vi "Find Time Zero.vi"() -> ()   [LabVIEW 2020]
uses:
  <vilib>/Analysis/1siggen.llb/Ramp Pattern by Samples.vi
  <vilib>/Analysis/NI_AALBase.lvlib
  SMC100-DQMH/Libraries/SMC100/SMC100.lvlib
  OphirPM-DQMH/Libraries/Ophir Power Meter/Ophir Power Meter.lvlib
panel:
  in  "Readout Rate (Hz)":i32=10
  in  "Ophir Port":i16=4
  in  "Power Range":u16(ring) items=["1.00mJ", "200uJ", "20.0uJ", "2.00uJ"]
  in  "SMC 100 Port":u8=3
  in  "Samples to Average":i32
  in  "Start Button":bool
  out "XY Graph":cluster{"Delay Positions":dbl[], "power":dbl[]}(graph)
  in  "Steps":i32
  in  "End Position":dbl
  in  "Start Posistion":dbl
  in  "OK":bool
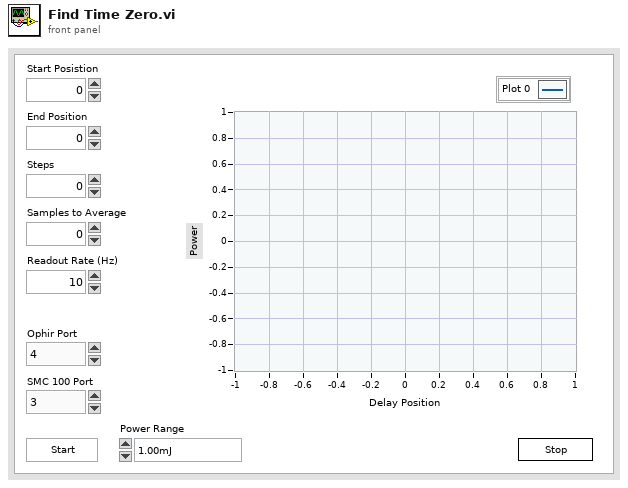
[diagram p1: front panel]
types:
  T1 = enum32{"Invalid", "Standard", "Closed", "Hidden", "Minimized", "Maximized"}
  T2 = enum32{"invalid app kind", "Development System", "Run Time System", "Student Edition", "Embedded LabVIEW", "Evaluation", "Custom"}
  T3 = cluster{"Core":cluster{"Current VI Reference":refnum<vi>, "Close Panel on Exit?":bool}, "Average":dbl[], "power":dbl[], "Delay Positions":dbl[], "Range Index":i32, "Step Index":i32}
  T4 = cluster{"Current VI Reference":refnum<vi>, "Close Panel on Exit?":bool}
  T5 = typedef "Ophir Power Meter.lvlib/Get Range Info (Reply Payload)--cluster.ctl" = cluster{"Range Info":cluster{"Strings Array":string[], "Symbols Array":i32[], "First Index":i32}, "Get Range Info_error":errorcluster}
  T6 = typedef "Ophir Power Meter.lvlib/Get Power Value (Reply Payload)--cluster.ctl" = cluster{"Power Value":dbl, "Get Power Value_error":errorcluster}
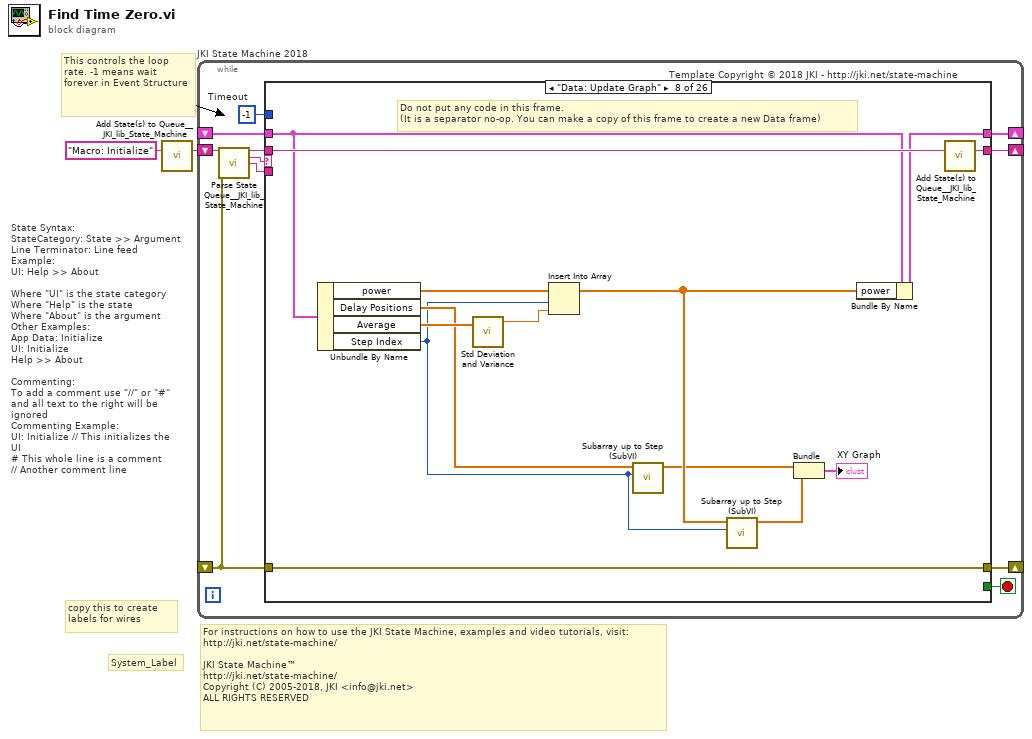
[diagram p0: block diagram]
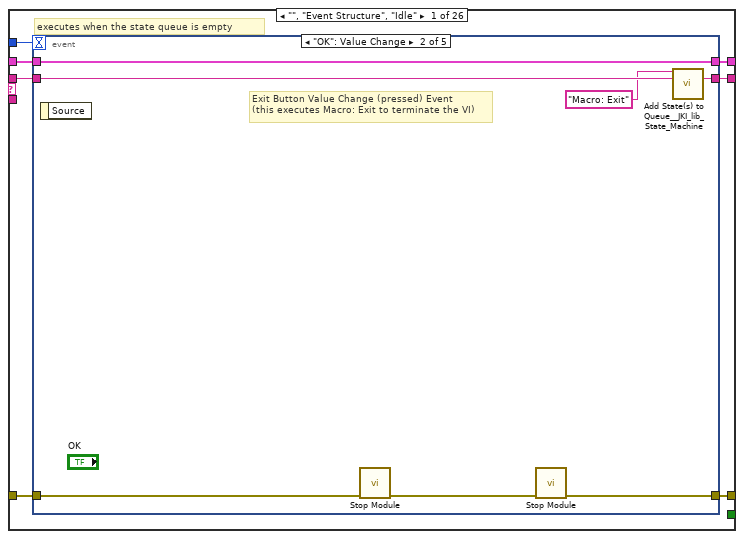
[diagram p2: hidden frame]
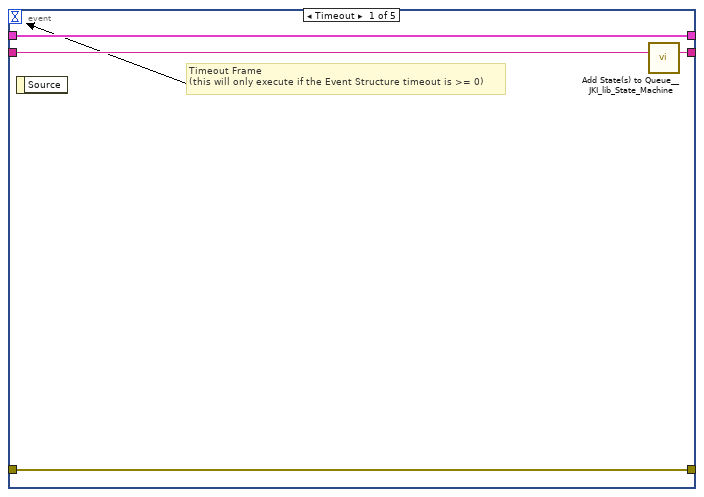
[diagram p3: hidden frame]
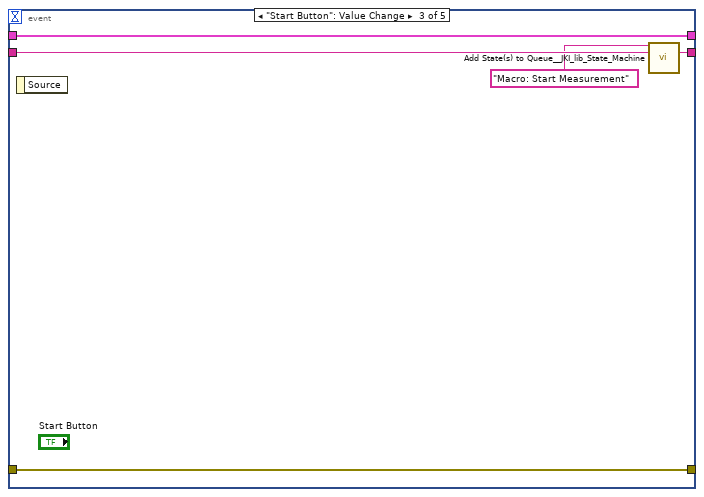
[diagram p4: hidden frame]
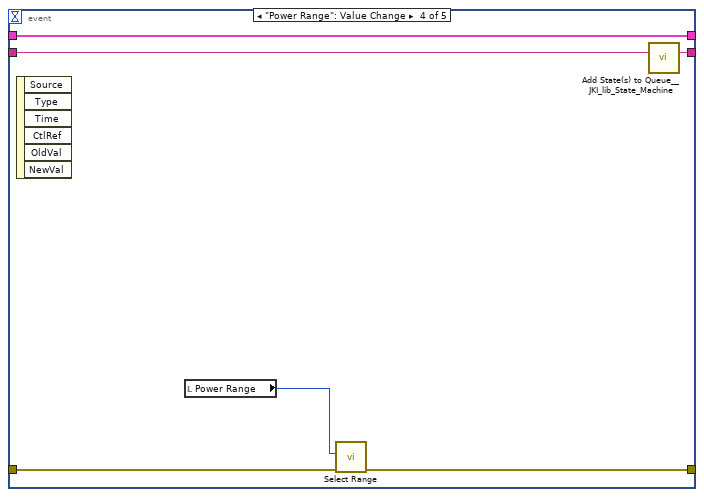
[diagram p5: hidden frame]
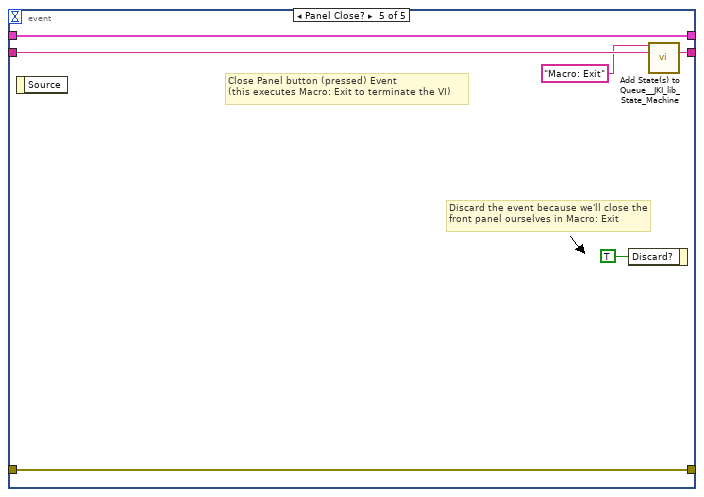
[diagram p6: hidden frame]
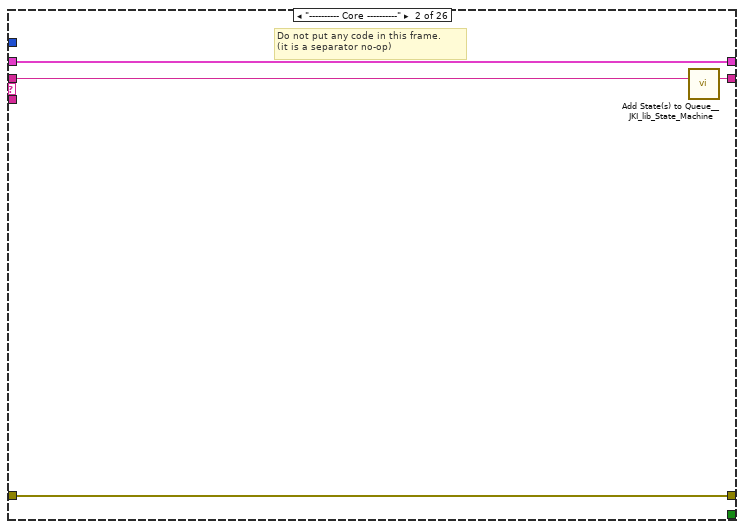
[diagram p7: hidden frame]
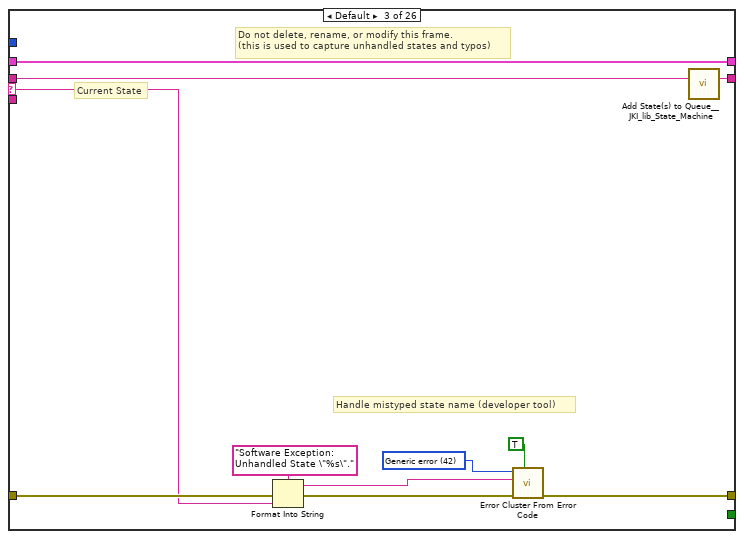
[diagram p8: hidden frame]
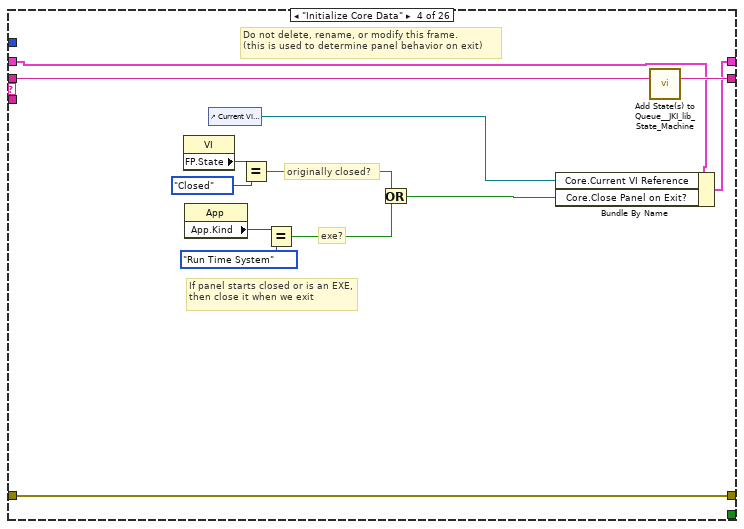
[diagram p9: hidden frame]
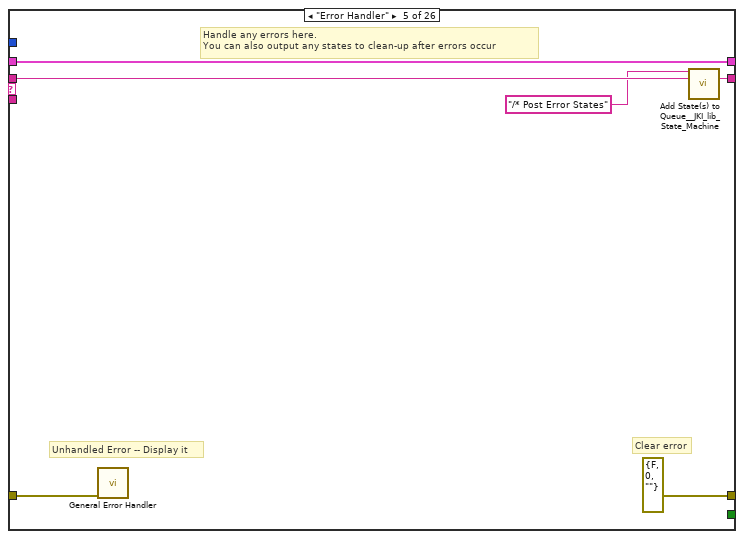
[diagram p10: hidden frame]
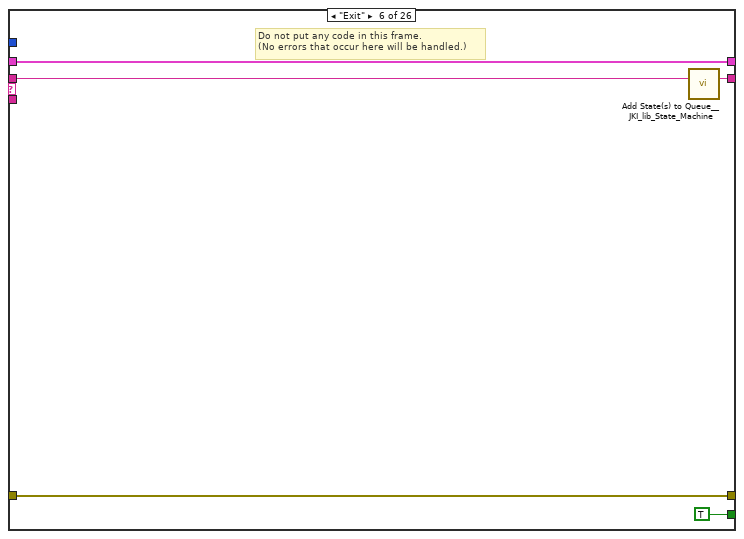
[diagram p11: hidden frame]
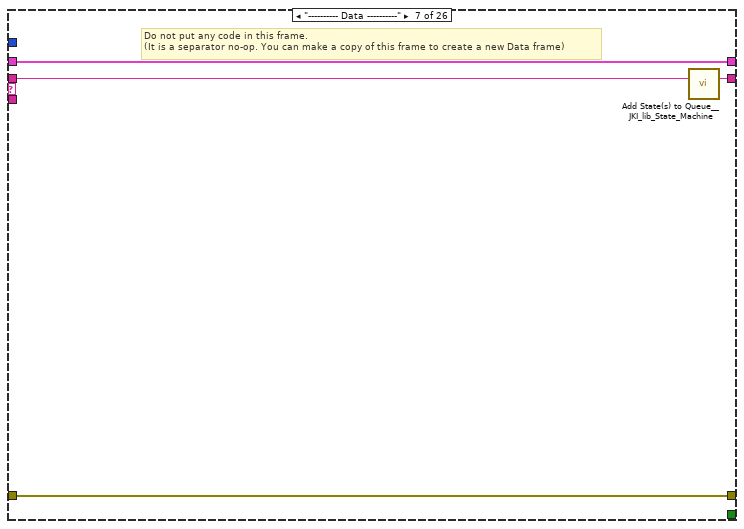
[diagram p12: hidden frame]
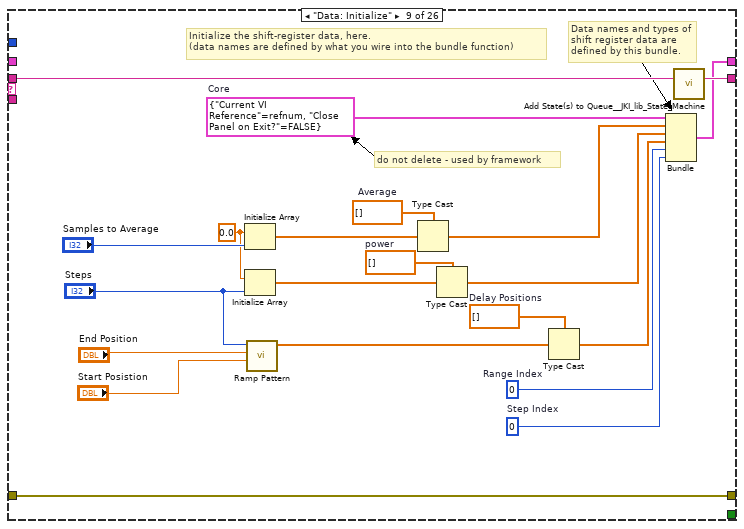
[diagram p13: hidden frame]
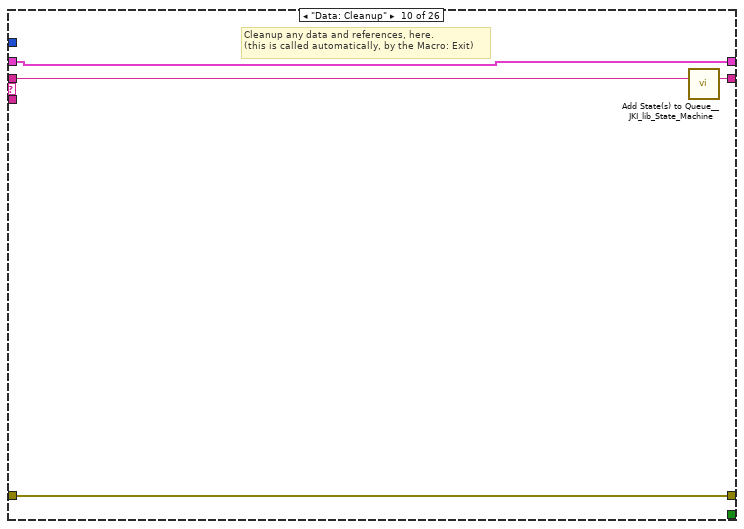
[diagram p14: hidden frame]
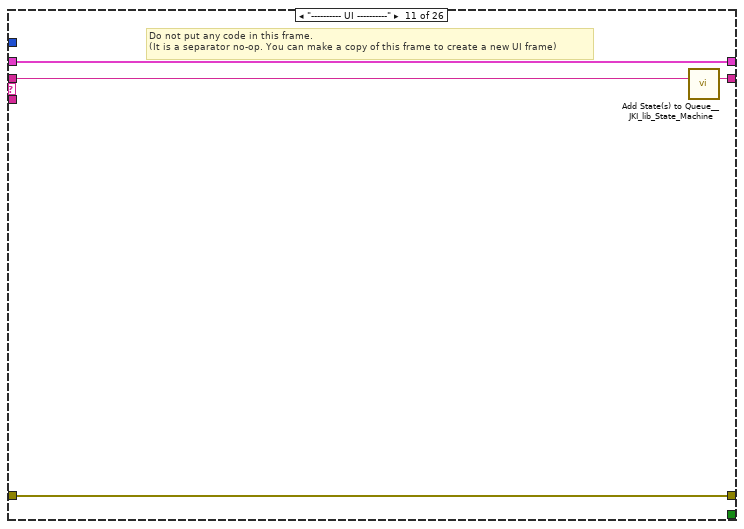
[diagram p15: hidden frame]
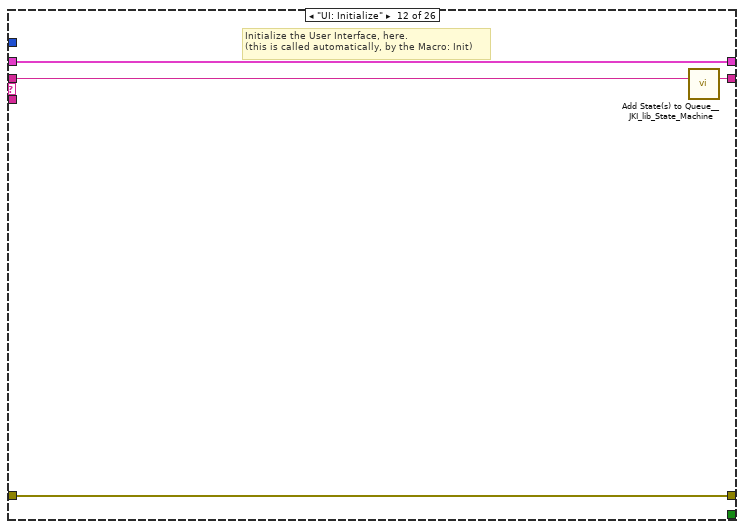
[diagram p16: hidden frame]
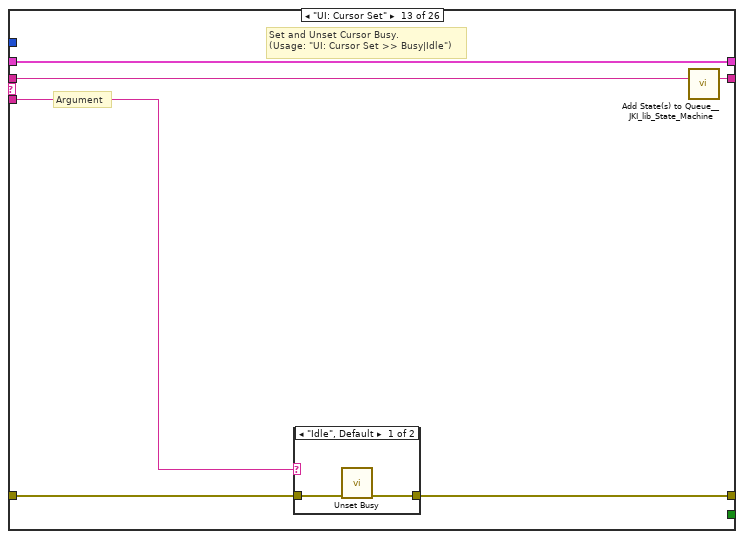
[diagram p17: hidden frame]
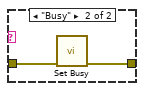
[diagram p18: hidden frame]
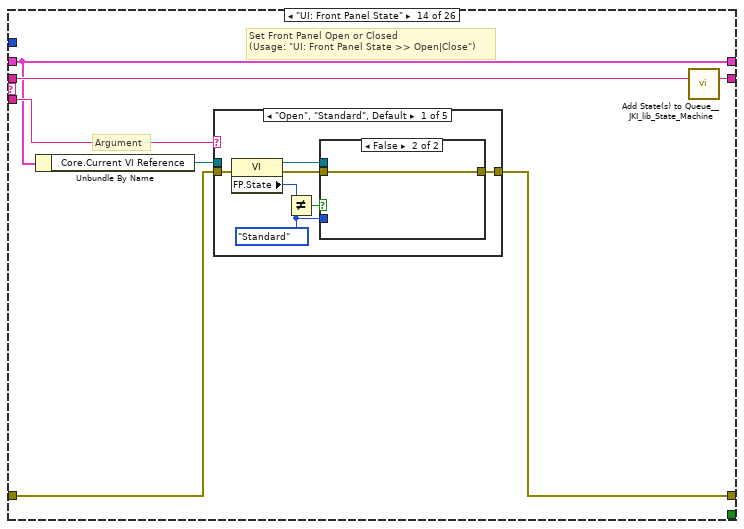
[diagram p19: hidden frame]
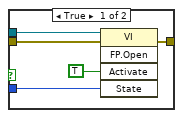
[diagram p20: hidden frame]
diagram:
  # "For instructions on how to use the JKI State Machine, examples and video tutorials, visit:\nhttp://jki.net/state-machine/\n\nJKI State Machine™\nhttp://jki.net/state-machine/\nCopyright (C) 2005-2018, JKI <info@jki.net>\nALL RIGHTS RESERVED"
  # "State Syntax:\nStateCategory: State >> Argument\nLine Terminator: Line feed\nExample:\nUI: Help >> About\n\nWhere \"UI\" is the state category\nWhere \"Help\" is the state\nWhere \"About\" is the argument\nOther Examples:\nApp Data: Initialize\nUI: Initialize\nHelp >> About\n\nCommenting:\nTo add a comment use \"//\" or \"#\" and all text to the right will be ignored\nCommenting Example:\nUI: Initialize // This initializes the UI\n# This whole line is a comment\n// Another comment line"
  # "copy this to create labels for wires"
  # "This controls the loop rate. -1 means wait forever in Event Structure"
  # "System_Label"
  n1 = call <vilib>:"Add State(s) to Queue__JKI_lib_State_Machine.vi"("State(s) in (\"\")"="Macro: Initialize") -> ("States Out"=w2:string)  [unwired: 14 in]
  n2 = while "JKI State Machine 2018" {
    shift-right: [w6] -> _
    shift-left: _ -> [w5]
    shift-right: [w9] -> _
    shift-left: _ -> [w3]
    shift-right: [w8] -> _
    shift-left: w2 -> [w10]
    stop <- w7 stop-if-true
    w4 = -1  # Timeout
    # "Template Copyright © 2018 JKI - http://jki.net/state-machine"
    n3 = call <vilib>:"Parse State Queue__JKI_lib_State_Machine.vi"("State Queue"=w10, "Error In (no error)"=w3) -> ("Remaining States"=w12:string, "Current State"=w13:string, "Arguments"=w11:string)  [unwired: 11 in]
    n4 = case shown="\"Data: Update Graph\"" w13 {
      selector: w13 -> [_ _ w53 _ _ _ _ _ _ _ _ _ _ _ _ _ _ _ _ _ _ _ _ _ _ _]
      tunnel: w12 -> [w20 w52 w57 w76 w82 w87 w91 w105 w126 w130 w134 w138 w144 w155 w219 w224 w229 w234 w244 w248 w255 w264 w274 w290 w308 w316]
      tunnel: w11 -> [_ _ _ _ _ _ _ _ _ _ _ _ w139 w150 _ _ _ _ _ _ _ _ _ _ _ _]
      tunnel: w5 -> [w18 w49 w55 w65 w79 w85 w88 w102 _ w127 w131 w136 w142 w149 w216 w221 w226 w231 w235 w245 w252 w261 w267 w288 w305 w312]
      tunnel: [w17 w50 w59 w74 errorcluster {"status"=FALSE, "code"=0, "source"=""} ("error out") w84 w89 w103 w124 w128 w132 w135 w140 w152 w217 w222 w227 w232 w242 w246 w251 w259 w272 w286 w304 w313] -> w9
      tunnel: w3 -> [w16 w50 w58 w74 w78 w84 w89 w103 w124 w128 w132 w135 w141 w153 w217 w222 w227 w232 w242 w246 w253 w262 w272 w287 w306 w314]
      tunnel: [w19 w51 w56 w75 w81 w86 w90 w104 w125 w129 w133 w137 w143 w154 w218 w223 w228 w233 w243 w247 w254 w263 w273 w289 w307 w315] -> w8
      tunnel: [_ _ _ _ _ TRUE _ _ _ _ _ _ _ _ _ _ _ _ _ _ _ _ _ _ _ _] -> w7
      tunnel: [w15 w49 w55 w64 w79 w85 w88 w101 w115 w127 w131 w136 w142 w149 w216 w221 w226 w231 w235 w245 w252 w261 w266 w288 w305 w312] -> w6
      tunnel: w4 -> [w14 _ _ _ _ _ _ _ _ _ _ _ _ _ _ _ _ _ _ _ _ _ _ _ _ _]
      frame "", "Event Structure", "Idle" {
        # "executes when the state queue is empty"
        n5 = event shown="[1] \"OK\": Value Change" {
          selector: _ -> [_ _ _ _ _]
          dyn-events: _ -> [_ _ _ _ _]
          timeout: w14 -> [_ _ _ _ _]
          tunnel: w20 -> [w24 w31 w36 w42 w48]
          tunnel: [w23 w30 w35 w41 w47] -> w19
          tunnel: w18 -> [w21 w28 w33 w39 w45]
          tunnel: [w22 w25 w34 w38 w46] -> w17
          tunnel: w16 -> [w22 w29 w34 w40 w46]
          tunnel: [w21 w28 w33 w39 w45] -> w15
          event Timeout {
            # "Timeout Frame\n(this will only execute if the Event Structure timeout is >= 0)"
            n6 = event-data() -> ()  [unwired: 1 in, 1 out]
            n7 = call <vilib>:"Add State(s) to Queue__JKI_lib_State_Machine.vi"("State(s) in (\"\")"=w24) -> ("States Out"=w23:string)  [unwired: 14 in]
          }
          event "OK": Value Change {
            # "Exit Button Value Change (pressed) Event\n(this executes Macro: Exit to terminate the VI)"
            n8 = event-data() -> ()  [unwired: 1 in, 1 out]
            n9 = call "Stop Module.vi"("error in (no error)"=w29) -> ("error out"=w26:errorcluster)  [unwired: 10 in]
            n10 = call "Stop Module.vi"("error in (no error)"=w26) -> ("error out"=w25:errorcluster)  [unwired: 10 in]
            n11 = call <vilib>:"Add State(s) to Queue__JKI_lib_State_Machine.vi"("State(s) in Front (\"\")"="Macro: Exit", "State(s) in (\"\")"=w31) -> ("States Out"=w30:string)  [unwired: 13 in]
          }
          event "Start Button": Value Change {
            n12 = event-data() -> ()  [unwired: 1 in, 1 out]
            n13 = call <vilib>:"Add State(s) to Queue__JKI_lib_State_Machine.vi"("State(s) in Front (\"\")"="Macro: Start Measurement", "State(s) in (\"\")"=w36) -> ("States Out"=w35:string)  [unwired: 13 in]
          }
          event "Power Range": Value Change {
            n14 = event-data() -> ()  [unwired: 1 in, 6 out]
            n15 = local read "Power Range"() -> (w37:u16)
            n16 = call "Select Range.vi"("error in (no error)"=w40, "Range Number"=w37) -> ("error out"=w38:errorcluster)  [unwired: 9 in]
            n17 = call <vilib>:"Add State(s) to Queue__JKI_lib_State_Machine.vi"("State(s) in (\"\")"=w42) -> ("States Out"=w41:string)  [unwired: 14 in]
          }
          event Panel Close? {
            # "Discard the event because we'll close the front panel ourselves in Macro: Exit"
            # "Close Panel button (pressed) Event\n(this executes Macro: Exit to terminate the VI)"
            n18 = event-data() -> ()  [unwired: 1 in, 1 out]
            n19 = event-data("Discard?"=TRUE) -> ()  [unwired: 1 in, 1 out]
            n20 = call <vilib>:"Add State(s) to Queue__JKI_lib_State_Machine.vi"("State(s) in Front (\"\")"="Macro: Exit", "State(s) in (\"\")"=w48) -> ("States Out"=w47:string)  [unwired: 13 in]
          }
        }
      }
      frame "---------- Core ----------" {
        # "Do not put any code in this frame.\n(it is a separator no-op)"
        n21 = call <vilib>:"Add State(s) to Queue__JKI_lib_State_Machine.vi"("State(s) in (\"\")"=w52) -> ("States Out"=w51:string)  [unwired: 14 in]
      }
      frame Default {
        w62 = 42 items=["No error", "Argument error", "Memory is full", "Out of zone", "End of file", "File already open", "Generic file I/O error", "File not found", "File permission error", "Disk is full", "Duplicate path", "Too many files open", "System feature not enabled", "Resource file not found", "Cannot add resource", "Resource not found", "Image not found", "Image memory error", "Pen does not exist", "Config type invalid", "Config token not found", "Config parse error", "Config memory error", "Bad external code format", "Bad external code offset", "External code not present", "Null window", "Destroy window error", "Null menu", "Print aborted", "Bad print record", "Print driver error", "Windows error during printing", "Memory error during printing", "Print dialog error", "Generic print error", "Invalid device refnum", "Device not found", "Device parameter error", "Device unit error", "Cannot open device", "Device call aborted", "Generic error", "Cancelled by user", "Object ID too low", "Object ID too high", "Object not in heap", "Unknown heap", "Unknown object (invalid DefProc)", "Unknown object (DefProc not in table)", "Message out of range", "Invalid (null) method", "Unknown message", "Manager call not supported", "Bad address", "Network operation in progress", "Network operation timed out", "Connection is busy", "Network attribute not supported", "Network error", "Address in use", "System out of memory", "Connection aborted", "Connection refused", "Not connected", "Already connected", "Connection closed", "Initialization error (interapplication manager)", "Bad occurrence", "Wait on unbound occurrence handler", "Occurrence queue overflow", "Datalog type conflict", "Unused", "Unrecognized type (interapplication manager)", "Memory corrupt", "Failed to make temporary DLL", "Old CIN version", "Drag socket not found", "Failed to load drop-object", "Failed to register OLE object", "Failed to release OLE object", "Format specifier type mismatch", "Unknown format specifier", "Too few format specifiers", "Too many format specifiers", "Scan failed", "Newer CIN version", "Error converting to variant", "Runtime menu error", "Password tampered", "Variant attribute not found", "Incompatible variant data type", "Event data is not available", "Event Store is not present", "Occurrence is not found", "Event Queue is not created", "Event info is not available", "Refnum passed is NULL", "Error retrieving Class GUID", "Error retrieving CoClass GUID", "Error retrieving TypeLib GUID.", "Bad built application magic bytes.", "Specific driver is different from the specific driver associated with the Logical Name.", "There is no session opened to the class driver.", "Max Error", "MAX - Error with config objects", "MAX - Error loading configuration", "MAX - Group not supported"]
        # "Current State"
        # "Do not delete, rename, or modify this frame.\n(this is used to capture unhandled states and typos)"
        # "Handle mistyped state name (developer tool)"
        n22 = Format Into String(format string="Software Exception: Unhandled State \"%s\"." ("message"), error in=w58, w53) -> (resulting string=w61:string, error out=w60:errorcluster)  [unwired: 1 in]
        n23 = call <vilib>:"Error Cluster From Error Code.vi"("show call chain? (False)"=TRUE, "error in (no error)"=w60, "error message (\"\")"=w61, "error code (0)"=w62) -> ("error out"=w59:errorcluster)  [unwired: 5 in]
        n24 = call <vilib>:"Add State(s) to Queue__JKI_lib_State_Machine.vi"("State(s) in (\"\")"=w57) -> ("States Out"=w56:string)  [unwired: 14 in]
      }
      frame "Initialize Core Data" {
        # "Do not delete, rename, or modify this frame.\n(this is used to determine panel behavior on exit)"
        # "originally closed?"
        # "exe?"
        # "If panel starts closed or is an EXE, then close it when we exit"
        n25 = property class="VI"() -> ("FP.State"=w68:T1)  [unwired: 2 in, 2 out]
        n26 = property class="App"() -> ("App.Kind"=w73:T2)  [unwired: 2 in, 2 out]
        n27 = control-ref of="Current VI Reference"() -> (w69:refnum<vi>)
        n28 = Equal?(x=w68, y=T1."Closed" ("Front Panel Window:State")) -> (x = y?=w66:bool)
        n29 = Equal?(x=w73, y=T2."Run Time System" ("Application:Kind")) -> (x = y?=w71:bool)
        n30 = Or(x=w66, y=w71) -> (x .or. y?=w70:bool)
        n31 = Bundle By Name(cluster=w65, "Core.Current VI Reference"=w69, "Core.Close Panel on Exit?"=w70) -> (w64:T3)
        n32 = call <vilib>:"Add State(s) to Queue__JKI_lib_State_Machine.vi"("State(s) in (\"\")"=w76) -> ("States Out"=w75:string)  [unwired: 14 in]
      }
      frame "Error Handler" {
        # "Unhandled Error -- Display it"
        # "Handle any errors here.\nYou can also output any states to clean-up after errors occur"
        # "Clear error"
        n33 = call <vilib>:"General Error Handler.vi"("error in (no error)"=w78) -> ()  [unwired: 10 in, 5 out]
        n34 = call <vilib>:"Add State(s) to Queue__JKI_lib_State_Machine.vi"("State(s) in Front (\"\")"="/* Post Error States", "State(s) in (\"\")"=w82) -> ("States Out"=w81:string)  [unwired: 13 in]
      }
      frame "Exit" {
        # "Do not put any code in this frame.\n(No errors that occur here will be handled.)"
        n35 = call <vilib>:"Add State(s) to Queue__JKI_lib_State_Machine.vi"("State(s) in (\"\")"=w87) -> ("States Out"=w86:string)  [unwired: 14 in]
      }
      frame "---------- Data ----------" {
        # "Do not put any code in this frame.\n(It is a separator no-op. You can make a copy of this frame to create a new Data frame)"
        n36 = call <vilib>:"Add State(s) to Queue__JKI_lib_State_Machine.vi"("State(s) in (\"\")"=w91) -> ("States Out"=w90:string)  [unwired: 14 in]
      }
      frame "Data: Update Graph" {
        # "Do not put any code in this frame.\n(It is a separator no-op. You can make a copy of this frame to create a new Data frame)"
        n37 = Unbundle By Name(w102) -> ("power"=w99:dbl[], "Delay Positions"=w96:dbl[], "Average"=w100:dbl[], "Step Index"=w92:i32)
        n38 = call <vilib>:"Std Deviation and Variance.vi"("X"=w100) -> ("mean"=w98:dbl)  [unwired: 1 in, 2 out]
        n39 = Insert Into Array(array=w99, index=w92, new element=w98) -> (w95:dbl[])
        n40 = call "Subarray up to Step (SubVI).vi"("Step Index"=w92, "Delay Positions"=w96) -> ("Array"=w94:dbl[])  [unwired: 9 in]
        n41 = call "Subarray up to Step (SubVI).vi"("Step Index"=w92, "Delay Positions"=w95) -> ("Array"=w93:dbl[])  [unwired: 9 in]
        n42 = Bundle("Array"=w94, "Array"=w93) -> (→"XY Graph":cluster{"Array":dbl[], "Array":dbl[]})  [unwired: 1 in]
        n43 = Bundle By Name(cluster=w102, "power"=w95) -> (w101:T3)
        n44 = call <vilib>:"Add State(s) to Queue__JKI_lib_State_Machine.vi"("State(s) in (\"\")"=w105) -> ("States Out"=w104:string)  [unwired: 14 in]
      }
      frame "Data: Initialize" {
        w106 = dbl[] []  # Delay Positions
        w108 = dbl[] []  # power
        w110 = dbl[] []  # Average
        w113 = 0  # Step Index
        w114 = 0  # Range Index
        w121 = 0.0 ("element")
        w123 = T4 {"Current VI Reference"=refnum, "Close Panel on Exit?"=FALSE}  # Core
        # "do not delete - used by framework"
        # "Data names and types of shift register data are defined by this bundle."
        # "Initialize the shift-register data, here.\n(data names are defined by what you wire into the bundle function)"
        n45 = Initialize Array(w121, "Samples to Average") -> (w112:dbl[])
        n46 = Initialize Array(w121, "Steps") -> (w120:dbl[])
        n47 = call-poly <vilib>:"Ramp Pattern.vi"("start"="Start Posistion", "end"="End Position", "samples"="Steps") -> ("Ramp Pattern"=w116:dbl[])  [unwired: 7 in, 1 out]
        n48 = Type Cast(type=w110, x=w112) -> (*(type *) &x=w111:dbl[])
        n49 = Type Cast(type=w108, x=w120) -> (*(type *) &x=w109:dbl[])
        n50 = Type Cast(type=w106, x=w116) -> (*(type *) &x=w107:dbl[])
        n51 = Bundle("Core"=w123, "Average"=w111, "power"=w109, "Delay Positions"=w107, "Range Index"=w114, "Step Index"=w113) -> (w115:T3)  [unwired: 1 in]
        n52 = call <vilib>:"Add State(s) to Queue__JKI_lib_State_Machine.vi"("State(s) in (\"\")"=w126) -> ("States Out"=w125:string)  [unwired: 14 in]
      }
      frame "Data: Cleanup" {
        # "Cleanup any data and references, here.\n(this is called automatically, by the Macro: Exit)"
        n53 = call <vilib>:"Add State(s) to Queue__JKI_lib_State_Machine.vi"("State(s) in (\"\")"=w130) -> ("States Out"=w129:string)  [unwired: 14 in]
      }
      frame "---------- UI ----------" {
        # "Do not put any code in this frame.\n(It is a separator no-op. You can make a copy of this frame to create a new UI frame)"
        n54 = call <vilib>:"Add State(s) to Queue__JKI_lib_State_Machine.vi"("State(s) in (\"\")"=w134) -> ("States Out"=w133:string)  [unwired: 14 in]
      }
      frame "UI: Initialize" {
        # "Initialize the User Interface, here.\n(this is called automatically, by the Macro: Init)"
        n55 = call <vilib>:"Add State(s) to Queue__JKI_lib_State_Machine.vi"("State(s) in (\"\")"=w138) -> ("States Out"=w137:string)  [unwired: 14 in]
      }
      frame "UI: Cursor Set" {
        # "Argument"
        # "Set and Unset Cursor Busy.\n(Usage: \"UI: Cursor Set >> Busy|Idle\")"
        n56 = case shown="\"Idle\", Default" w139 {
          tunnel: w141 -> [w146 w148]
          tunnel: [w145 w147] -> w140
          frame "Idle", Default {
            n57 = call <vilib>:"Unset Busy.vi"("error in (no error)"=w146) -> ("error out"=w145:errorcluster)  [unwired: 10 in]
          }
          frame "Busy" {
            n58 = call <vilib>:"Set Busy.vi"("error in (no error)"=w148) -> ("error out"=w147:errorcluster)  [unwired: 9 in, 1 out]
          }
        }
        n59 = call <vilib>:"Add State(s) to Queue__JKI_lib_State_Machine.vi"("State(s) in (\"\")"=w144) -> ("States Out"=w143:string)  [unwired: 14 in]
      }
      frame "UI: Front Panel State" {
        # "Argument"
        # "Set Front Panel Open or Closed\n(Usage: \"UI: Front Panel State >> Open|Close\")"
        n60 = Unbundle By Name(w149) -> ("Core.Current VI Reference"=w151:refnum<vi>)
        n61 = case shown="\"Open\", \"Standard\", Default" w150 {
          tunnel: w153 -> [w161 w174 w185 w197 w209]
          tunnel: [w162 w175 w186 w198 w210] -> w152
          tunnel: w151 -> [_ _ _ _ _]
          frame "Open", "Standard", Default {
            w156 = T1."Standard" ("State")
            n62 = property class="VI"(error in=w161) -> (reference out=w159:refnum<vi>, error out=w160:errorcluster, "FP.State"=w158:T1)  [unwired: 1 in]
            n63 = Not Equal?(x=w158, y=w156) -> (x != y?=w157:bool)
            n64 = case shown="False" w157 {
              tunnel: [w166 w168] -> w162
              tunnel: w160 -> [w165 w168]
              tunnel: w159 -> [w164 _]
              tunnel: w156 -> [w163 _]
              frame True {
                n65 = invoke class="VI" method="FP.Open"(reference=w164, error in=w165, "Activate"=TRUE, "State"=w163) -> (error out=w166:errorcluster)  [unwired: 1 in, 4 out]
              }
              frame False {
              }
            }
          }
          frame "Close", "Closed" {
            n66 = property class="VI"(error in=w174) -> (reference out=w172:refnum<vi>, error out=w173:errorcluster, "FP.State"=w170:T1)  [unwired: 1 in]
            n67 = Not Equal?(x=w170, y=T1."Closed" ("Front Panel Window:State")) -> (x != y?=w169:bool)
            n68 = case shown="True" w169 {
              tunnel: [w176 w179] -> w175
              tunnel: w173 -> [w176 w178]
              tunnel: w172 -> [_ w177]
              frame False {
              }
              frame True {
                n69 = invoke class="VI" method="FP.Close"(reference=w177, error in=w178) -> (error out=w179:errorcluster)  [unwired: 1 in, 2 out]
              }
            }
          }
          frame "Hidden", "Hide" {
            w180 = T1."Hidden" ("State")
            n70 = property class="VI"(error in=w185) -> (reference out=w183:refnum<vi>, error out=w184:errorcluster, "FP.State"=w182:T1)  [unwired: 1 in]
            n71 = Not Equal?(x=w182, y=w180) -> (x != y?=w181:bool)
            n72 = case shown="True" w181 {
              tunnel: [w190 w191] -> w186
              tunnel: w184 -> [w189 w191]
              tunnel: w183 -> [w188 _]
              tunnel: w180 -> [w187 _]
              frame True {
                n73 = invoke class="VI" method="FP.Open"(reference=w188, error in=w189, "State"=w187) -> (error out=w190:errorcluster)  [unwired: 2 in, 4 out]
              }
              frame False {
              }
            }
          }
          frame "Minimize", "Minimized" {
            w192 = T1."Minimized" ("State")
            n74 = property class="VI"(error in=w197) -> (reference out=w195:refnum<vi>, error out=w196:errorcluster, "FP.State"=w194:T1)  [unwired: 1 in]
            n75 = Not Equal?(x=w194, y=w192) -> (x != y?=w193:bool)
            n76 = case shown="True" w193 {
              tunnel: [w202 w203] -> w198
              tunnel: w196 -> [w201 w203]
              tunnel: w195 -> [w200 _]
              tunnel: w192 -> [w199 _]
              frame True {
                n77 = invoke class="VI" method="FP.Open"(reference=w200, error in=w201, "State"=w199) -> (error out=w202:errorcluster)  [unwired: 2 in, 4 out]
              }
              frame False {
              }
            }
          }
          frame "Maximize", "Maximized" {
            w204 = T1."Maximized" ("State")
            n78 = property class="VI"(error in=w209) -> (reference out=w207:refnum<vi>, error out=w208:errorcluster, "FP.State"=w206:T1)  [unwired: 1 in]
            n79 = Not Equal?(x=w206, y=w204) -> (x != y?=w205:bool)
            n80 = case shown="True" w205 {
              tunnel: [w214 w215] -> w210
              tunnel: w208 -> [w213 w215]
              tunnel: w207 -> [w212 _]
              tunnel: w204 -> [w211 _]
              frame True {
                n81 = invoke class="VI" method="FP.Open"(reference=w212, error in=w213, "State"=w211) -> (error out=w214:errorcluster)  [unwired: 2 in, 4 out]
              }
              frame False {
              }
            }
          }
        }
        n82 = call <vilib>:"Add State(s) to Queue__JKI_lib_State_Machine.vi"("State(s) in (\"\")"=w155) -> ("States Out"=w154:string)  [unwired: 14 in]
      }
      frame "---------- Macro ----------" {
        # "Do not put any code in this frame.\n(It is a separator no-op. You can make a copy of this frame to create a new Macro frame)"
        n83 = call <vilib>:"Add State(s) to Queue__JKI_lib_State_Machine.vi"("State(s) in (\"\")"=w219) -> ("States Out"=w218:string)  [unwired: 14 in]
      }
      frame "Macro: Measurement Cycle" {
        # "Do not put any code in this frame.\n(It is a separator no-op. You can make a copy of this frame to create a new Macro frame)"
        n84 = call <vilib>:"Add State(s) to Queue__JKI_lib_State_Machine.vi"("State(s) in (\"\")"=w224, "State(s) at Back (\"\")"="Devices: Move to Position\nDevices: Get Average Power\nData: Update Graph\nDevices: Finished?" ("State(s) at Back (\"\")")) -> ("States Out"=w223:string)  [unwired: 13 in]
      }
      frame "Macro: Start Measurement" {
        # "Do not put any code in this frame.\n(It is a separator no-op. You can make a copy of this frame to create a new Macro frame)"
        n85 = call <vilib>:"Add State(s) to Queue__JKI_lib_State_Machine.vi"("State(s) in (\"\")"=w229, "State(s) at Back (\"\")"="Data: Initialize\nDevices: Initialize\nMacro: Measurement Cycle" ("State(s) at Back (\"\")")) -> ("States Out"=w228:string)  [unwired: 13 in]
      }
      frame "Macro: Initialize" {
        # "Initialization Macro\n(This is called once, when the VI starts)"
        n86 = call <vilib>:"Add State(s) to Queue__JKI_lib_State_Machine.vi"("State(s) in Front (\"\")"="Devices: Start\nData: Initialize\nInitialize Core Data\nUI: Initialize\nUI: Front Panel State >> Open\nDevices: Get Ranges", "State(s) in (\"\")"=w234) -> ("States Out"=w233:string)  [unwired: 13 in]
      }
      frame "Macro: Exit" {
        # "Exit Macro\n(This is called once, when the VI exits)"
        n87 = Unbundle By Name(w235) -> ("Core.Close Panel on Exit?"=w236:bool)
        n88 = Select(t="UI: Front Panel State >> Close", s=w236, f="") -> (s? t:f=w239:string)
        n89 = call <vilib>:"Add State(s) to Queue__JKI_lib_State_Machine.vi"("State(s) in (\"\")"=w239, "State(s) at Back (\"\")"="Data: Cleanup\nExit") -> ("States Out"=w237:string)  [unwired: 13 in]
        n90 = call <vilib>:"Add State(s) to Queue__JKI_lib_State_Machine.vi"("State(s) in Front (\"\")"=w237, "State(s) in (\"\")"=w244) -> ("States Out"=w243:string)  [unwired: 13 in]
      }
      frame "---------- Devices ----------" {
        # "Template Separator\n(You can make a copy of, or modify, this frame)"
        n91 = call <vilib>:"Add State(s) to Queue__JKI_lib_State_Machine.vi"("State(s) in (\"\")"=w248) -> ("States Out"=w247:string)  [unwired: 14 in]
      }
      frame "Devices: Get Ranges" {
        # "Template Separator\n(You can make a copy of, or modify, this frame)"
        n92 = call "Get Range Info.vi"("error in (no error)"=w253) -> ("error out"=w251:errorcluster, "Reply Payload"=w250:T5)  [unwired: 8 in, 1 out]
        n93 = Unbundle By Name(w250) -> ("Range Info.Strings Array"=w249:string[])
        n94 = property on="Power Range" class="Ring (strict)"("Strings []"=w249) -> ()  [unwired: 2 in, 2 out]
        n95 = call <vilib>:"Add State(s) to Queue__JKI_lib_State_Machine.vi"("State(s) in (\"\")"=w255) -> ("States Out"=w254:string)  [unwired: 14 in]
      }
      frame "Devices: Start" {
        # "Give devices time to initialize"
        # "Template Separator\n(You can make a copy of, or modify, this frame)"
        n96 = call "Start Module.vi"("error in (no error)"=w262, "Port Number"="Ophir Port") -> ("error out"=w260:errorcluster)  [unwired: 6 in, 3 out]
        n97 = Wait (ms)(milliseconds to wait=u32 2000) -> ()  [unwired: 1 out]
        n98 = call "Start Module.vi"("error in (no error)"=w260, "SerialPort"="SMC 100 Port") -> ("error out"=w259:errorcluster)  [unwired: 6 in, 3 out]
        n99 = call <vilib>:"Add State(s) to Queue__JKI_lib_State_Machine.vi"("State(s) in (\"\")"=w264) -> ("States Out"=w263:string)  [unwired: 14 in]
      }
      frame "Devices: Finished?" {
        # "Template Separator\n(You can make a copy of, or modify, this frame)"
        n100 = local read "Steps"() -> (w271:i32)
        n101 = Unbundle By Name(w267) -> ("Step Index"=w265:i32)
        n102 = Decrement(x=w271) -> (x-1=w270:i32)
        n103 = Greater Or Equal?(x=w265, y=w270) -> (x >= y?=w269:bool)
        n104 = case shown="False" w269 {
          tunnel: ["Macro: Measurement Cycle" ("State(s) at Back (\"\")") "Devices: Initialize" ("State(s) at Back (\"\")")] -> w268
          tunnel: w267 -> [w279 w282]
          tunnel: [w277 w281] -> w266
          tunnel: w265 -> [w276 _]
          frame False {
            n105 = Increment(x=w276) -> (x+1=w275:i32)
            n106 = Bundle By Name(cluster=w279, "Step Index"=w275) -> (w277:T3)
          }
          frame True {
            n107 = Bundle By Name(cluster=w282, "Step Index"=0) -> (w281:T3)
          }
        }
        n108 = call <vilib>:"Add State(s) to Queue__JKI_lib_State_Machine.vi"("State(s) in (\"\")"=w274, "State(s) at Back (\"\")"=w268) -> ("States Out"=w273:string)  [unwired: 13 in]
      }
      frame "Devices: Get Average Power" {
        # "Template Separator\n(You can make a copy of, or modify, this frame)"
        n109 = Unbundle By Name(w288) -> ("Average"=w285:dbl[])
        n110 = local read "Samples to Average"() -> (w284:i32)
        n111 = for {
          N: w284 -> [_]
          tunnel: [w301] -> w286
          tunnel: w287 -> [w302]
          shift-right: [w298] -> _
          shift-left: w285 -> [w299]
          i -> [w297]
          n112 = call "Get Power Value.vi"("error in (no error)"=w302) -> ("error out"=w301:errorcluster, "Reply Payload"=w300:T6)  [unwired: 8 in, 1 out]
          n113 = Unbundle By Name(w300) -> ("Power Value"=w296:dbl)
          n114 = Divide(x=1, y="Readout Rate (Hz)") -> (x/y=w293:dbl)
          n115 = Multiply(x=w293, y=1000.0) -> (x*y=w291:dbl)
          n116 = Insert Into Array(array=w299, index=w297, new element=w296) -> (w298:dbl[])
          n117 = Wait (ms)(milliseconds to wait=w291) -> ()  [unwired: 1 out]
        }
        n118 = call <vilib>:"Add State(s) to Queue__JKI_lib_State_Machine.vi"("State(s) in (\"\")"=w290) -> ("States Out"=w289:string)  [unwired: 14 in]
      }
      frame "Devices: Initialize" {
        # "Your code here.\n(You can make a copy of, or modify, this frame)"
        n119 = local read "Start Posistion"() -> (w303:dbl)
        n120 = call "Set Abs Position.vi"("error in (no error)"=w306, "Abolute Position"=w303) -> ("error out"=w304:errorcluster)  [unwired: 9 in]
        n121 = call <vilib>:"Add State(s) to Queue__JKI_lib_State_Machine.vi"("State(s) in (\"\")"=w308) -> ("States Out"=w307:string)  [unwired: 14 in]
      }
      frame "Devices: Move to Position" {
        # "Your code here.\n(You can make a copy of, or modify, this frame)"
        n122 = Unbundle By Name(w312) -> ("Delay Positions"=w311:dbl[], "Step Index"=w310:i32)
        n123 = Index Array(array=w311, index=w310) -> (element=w309:dbl)
        n124 = call "Set Abs Position.vi"("error in (no error)"=w314, "Abolute Position"=w309) -> ("error out"=w313:errorcluster)  [unwired: 9 in]
        n125 = call <vilib>:"Add State(s) to Queue__JKI_lib_State_Machine.vi"("State(s) in (\"\")"=w316) -> ("States Out"=w315:string)  [unwired: 14 in]
      }
    }
  }
